vi "Initialize Tree.vi"(11 "UI Data in":refnum<class "Settings UI.lvclass">) -> (3 "UI Data out":refnum<class "Settings UI.lvclass">)   [LabVIEW 2020, in "Output Sequencer.lvlib" / "Settings UI.lvclass"]
uses:
  Settings UI.lvclass
  Types/UI State.ctl
  <vilib>/Utility/miscctls.llb/LVNodeAndColumnTypeDef.ctl
  Types/Drag-Drop State.ctl
  Settings UI.lvclass/Settings UI.ctl
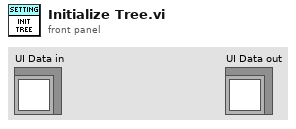
[diagram p1: front panel]
types:
  T1 = typedef "Output Sequencer.lvlib/Settings UI.lvclass/UI State.ctl" = cluster{"Pending Changes":bool, "Previous Tree Value":string, "Top Left":T2, "Drag-Drop State":T3}
  T2 = typedef "LVNodeAndColumnTypeDef.ctl" = cluster{"Node":string, "Column":i32}
  T3 = typedef "Output Sequencer.lvlib/Settings UI.lvclass/Drag-Drop State.ctl" = cluster{"Step Number":i32, "Current Index":i32, "Dropped?":bool, "Previous Open State":bool[]}
  T4 = cluster{"Left Cell String":string, "Child Text":string[], "Child Tag":string, "Item Indent":i32, "Child Only?":bool, "Glyph Index":i32}[]
  T5 = cluster{"Left Cell String":string, "Child Text":string[], "Child Tag":string, "Item Indent":i32, "Child Only?":bool, "Glyph Index":i32}
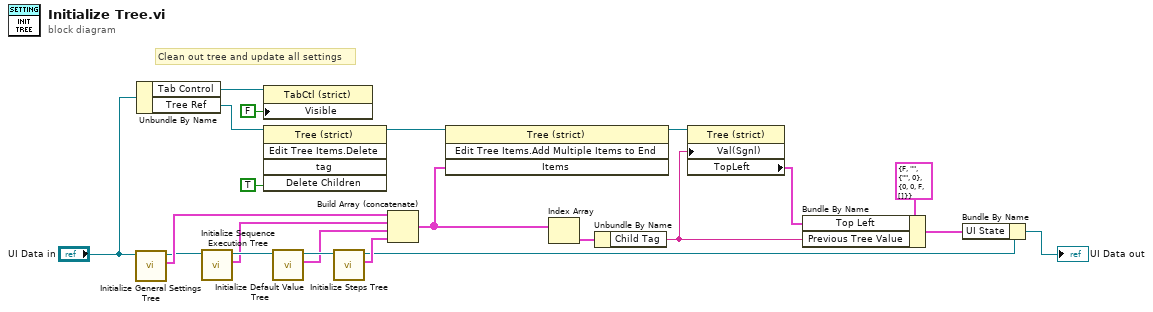
[diagram p0: block diagram]
diagram:
  # "Clean out tree and update all settings"
  n1 = call "Initialize General Settings Tree.vi"("UI Data in"="UI Data in") -> ("Items to Add"=w6:T4, "UI Data out"=w5:refnum<class "Settings UI.lvclass">)  [unwired: 9 in]
  n2 = Unbundle By Name("UI Data in") -> ("Tab Control"=w13:refnum<vi>, "Tree Ref"=w15:refnum<vi>)
  n3 = call "Initialize Sequence Execution Tree.vi"("UI Data in"=w5) -> ("Items to Add"=w7:T4, "UI Data out"=w8:refnum<class "Settings UI.lvclass">)  [unwired: 9 in]
  n4 = property class="TabCtl (strict)"(reference=w13, "Visible"=FALSE) -> ()  [unwired: 1 in, 2 out]
  n5 = invoke class="Tree (strict)" method="Edit Tree Items.Delete"(reference=w15, "Delete Children"=TRUE ("Delete Children?")) -> (reference out=w22:refnum<vi>)  [unwired: 3 in, 4 out]
  n6 = call "Initialize Default Value Tree.vi"("UI Data in"=w8) -> ("Items to Add"=w9:T4, "UI Data out"=w10:refnum<class "Settings UI.lvclass">)  [unwired: 9 in]
  n7 = call "Initialize Steps Tree.vi"("UI Data in"=w10) -> ("Items to Add"=w11:T4, "UI Data out"=w3:refnum<class "Settings UI.lvclass">)  [unwired: 9 in]
  n8 = Build Array (concatenate)(w6, w7, w9, w11) -> (w21:T4)
  n9 = invoke class="Tree (strict)" method="Edit Tree Items.Add Multiple Items to End"(reference=w22, "Items"=w21) -> (reference out=w19:refnum<vi>)  [unwired: 2 in, 3 out]
  n10 = Index Array(array=w21) -> (element=w20:T5)  [unwired: 1 in]
  n11 = Unbundle By Name(w20) -> ("Child Tag"=w16:string)
  n12 = property class="Tree (strict)"(reference=w19, "Val(Sgnl)"=w16) -> ("TopLeft"=w17:T2)  [unwired: 1 in, 2 out]
  n13 = Bundle By Name(cluster=T1 {"Pending Changes"=FALSE, "Previous Tree Value"="", "Top Left"={"Node"="", "Column"=0}, "Drag-Drop State"={"Step Number"=0, "Current Index"=0, "Dropped?"=FALSE, "Previous Open State"=[]}} ("Settings State"), "Top Left"=w17, "Previous Tree Value"=w16) -> (w2:T1)
  n14 = Bundle By Name(cluster=w3, "UI State"=w2) -> (→"UI Data out":refnum<class "Settings UI.lvclass">)
